vi "Create.vi"(9 "Alias":string, 10 "Nest Actor":refnum<class "LVCAM.lvclass">, 11 "Self Actor in":refnum<class "Self Actor.lvclass">) -> (0 "error out":errorcluster, 3 "Self Actor out":refnum<class "Self Actor.lvclass">)   [LabVIEW 2021, in "AAM.lvlib" / "Self Actor.lvclass"]
uses:
  Self Actor.lvclass
  C:/PPLs/LabVIEW-Composed-Actor-Model-LVCAM/LabVIEW-Composed-Actor-Model-LVCAM/AAM/AAM/LVCAM/LVCAM.lvclass
  LVCAM/LVCAM.lvclass
  Self Actor.lvclass/Self Actor.ctl
  LVCAM/Msg Loop.vi
  Msg Q/Msg Q.lvclass
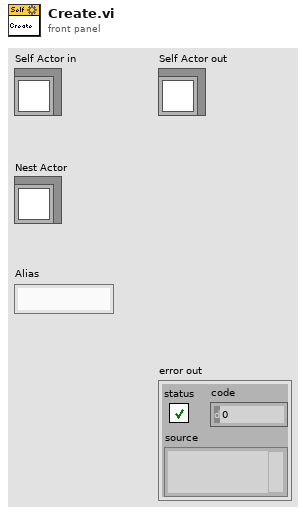
[diagram p1: front panel]
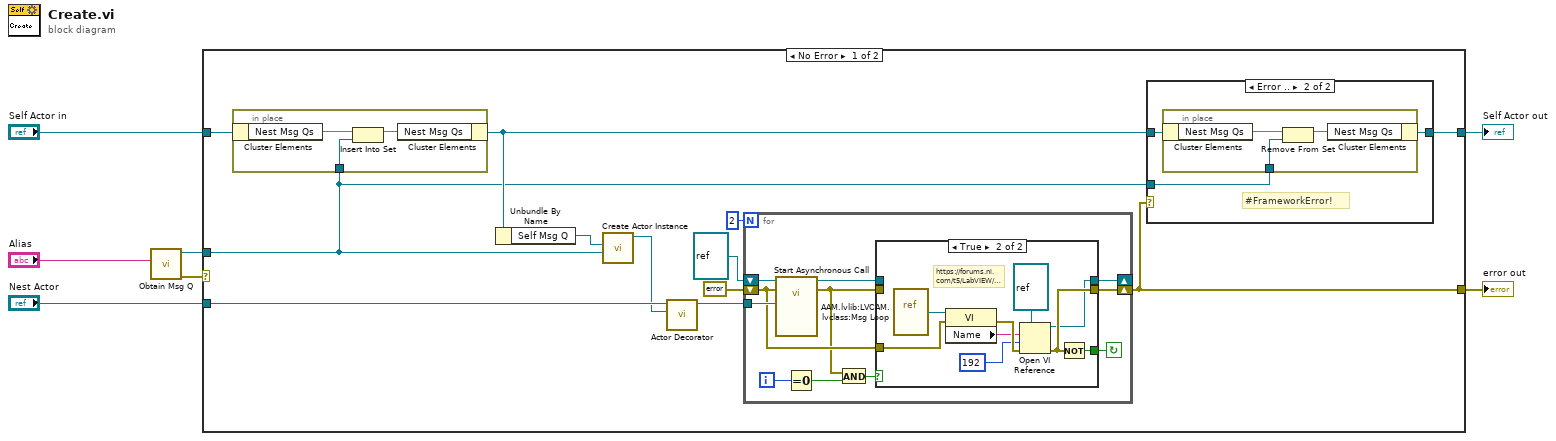
[diagram p0: block diagram]
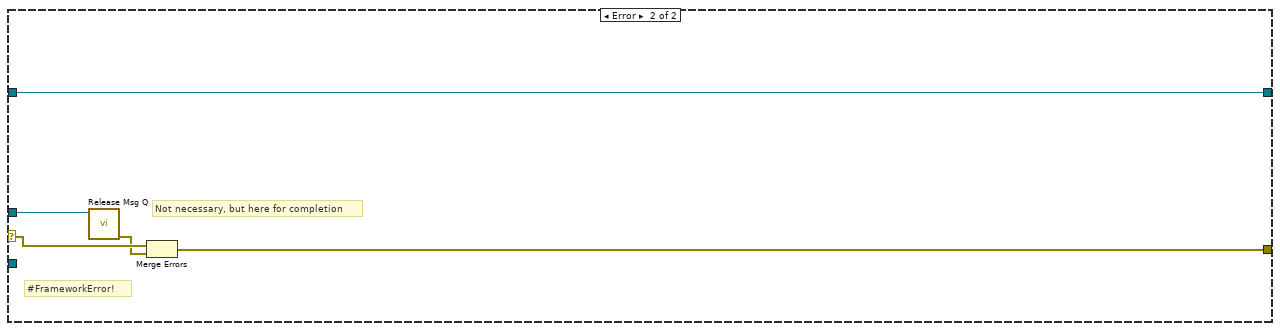
[diagram p4: hidden frame]
diagram:
  n1 = call "Obtain Msg Q.vi"("Alias"="Alias") -> ("error out"=w1:errorcluster, "Msg Queue out"=w2:refnum<class "Msg Q.lvclass">)  [unwired: 9 in]
  n2 = case shown="No Error" w1 {
    selector: w1 -> [_ w56]
    tunnel: "Self Actor in" -> [w19 w55]
    tunnel: [w15 w55] -> w5
    tunnel: [w16 w53] -> w4
    tunnel: "Nest Actor" -> [w10 _]
    tunnel: w2 -> [w11 w54]
    frame No Error {
      n3 = in-place {
        in-place-border: w11 -> [w49]
        n4 = in-place-cluster #1(w19) -> ("Nest Msg Qs"=w51:set{refnum<class "Msg Q.lvclass">})
        n5 = Insert Into Set(10:w49, 11:w51) -> (3:w50:set{refnum<class "Msg Q.lvclass">})  [unwired: 1 out]
        n6 = in-place-cluster #1("Nest Msg Qs"=w50) -> (w14:refnum<class "Self Actor.lvclass">)
      }
      n7 = Unbundle By Name(w14) -> ("Self Msg Q"=w12:refnum<class "Msg Q.lvclass">)
      n8 = call "Create Actor Instance.vi"("Self Msg Q"=w11, "Call Msg Q"=w12) -> ("Self Actor out"=w8:refnum<class "Self Actor.lvclass">)  [unwired: 9 in]
      n9 = call-dynamic "Actor Decorator.vi"("Actor"=w8, "Write Actor in"=w10) -> ("Write Actor out"=w9:refnum<class "LVCAM.lvclass">)  [unwired: 9 in]
      n10 = for {
        N: 2 -> [_]
        tunnel: w9 -> [w37]
        shift-right: [w28] -> w16
        shift-left: errorcluster {"status"=FALSE, "code"=0, "source"=""} ("error out") -> [w31]
        shift-right: [w34] -> _
        shift-left: refnum<vi> refnum ("type specifier VI Refnum (for type only)") -> [w27]
        i -> [w36]
        stop <- w30 continue-if-true
        n11 = call-by-ref "Start Asynchronous Call"(reference=w27, error in=w31, "Actor in"=w37) -> (reference out=w33:refnum<vi>, error out=w29:errorcluster)  [unwired: 11 in]
        n12 = Equal To 0?(x=w36) -> (x = 0?=w35:bool)
        n13 = And(x=w29, y=w35) -> (x .and. y?=w32:bool)
        n14 = case shown="True" w32 {
          tunnel: [w38 w43] -> w34
          tunnel: w33 -> [w38 _]
          tunnel: w31 -> [_ w47]
          tunnel: w29 -> [w39 _]
          tunnel: [_ w48] -> w30
          tunnel: [w39 w44] -> w28
          frame False {
          }
          frame True {
            # "https://forums.ni.com/t5/LabVIEW/Static-VI-Reference/m-p/3334014#M978333"
            n15 = vi-ref "AAM.lvlib:LVCAM.lvclass:Msg Loop.vi"() -> (w40:refnum<vi>)
            n16 = property class="VI"(reference=w40, error in=w47) -> (error out=w46:errorcluster, "Name"=w45:string)  [unwired: 1 out]
            n17 = Open VI Reference(type specifier VI Refnum (for type only)=refnum<vi> refnum, vi path=w45, options=192 ("options: Multiple Clones,\n  Fire & Forget"), error in (no error)=w46) -> (vi reference=w43:refnum<vi>, error out=w44:errorcluster)  [unwired: 2 in]
            n18 = Not(x=w44) -> (.not. x?=w48:bool)
          }
        }
      }
      n19 = case shown="Error .." w16 {
        tunnel: w14 -> [w20 w23]
        tunnel: [w20 w22] -> w15
        tunnel: w11 -> [_ w21]
        frame No Error {
        }
        frame Error {
          # "#FrameworkError!"
          n20 = in-place {
            in-place-border: w21 -> [w24]
            n21 = in-place-cluster #2(w23) -> ("Nest Msg Qs"=w26:set{refnum<class "Msg Q.lvclass">})
            n22 = Remove From Set(10:w24, 11:w26) -> (3:w25:set{refnum<class "Msg Q.lvclass">})  [unwired: 1 out]
            n23 = in-place-cluster #2("Nest Msg Qs"=w25) -> (w22:refnum<class "Self Actor.lvclass">)
          }
        }
      }
    }
    frame Error {
      # "#FrameworkError!"
      # "Not necessary, but here for completion"
      n24 = call "Release Msg Q.vi"("Msg Queue in"=w54) -> ("error out"=w52:errorcluster)  [unwired: 9 in, 1 out]
      n25 = Merge Errors(w56, w52) -> (w53:errorcluster)
    }
  }
  "error out" <- w4
  "Self Actor out" <- w5
